vi "Curvature of Bezier Spline.vi"(10 "percision":dbl=0.01, 11 "bezier spline waypts":T1) -> (3 "curvature":dbl[][](array[numeric]))   [LabVIEW 2019]
uses:
  Types/Bezier Spline.ctl
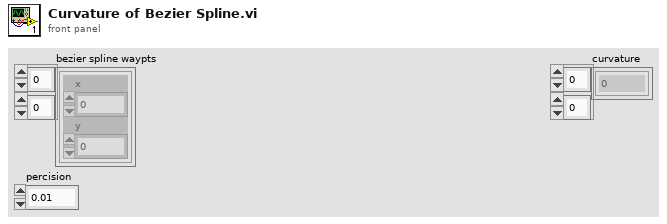
[diagram p1: front panel]
types:
  T1 = typedef "Bezier Spline.ctl" = cluster{"x":dbl, "y":dbl}[][]
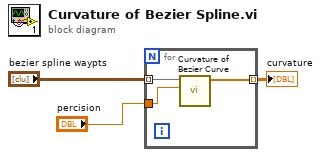
[diagram p0: block diagram]
diagram:
  n1 = for {
    tunnel: "bezier spline waypts" -> [w6] mode=indexing
    tunnel: [w5] -> w1 mode=indexing
    tunnel: "percision" -> [w4]
    n2 = call "Curvature of Bezier Curve.vi"("percision"=w4, "ctrl points"=w6) -> ("curvature"=w5:dbl[])  [unwired: 9 in]
  }
  "curvature" <- w1
